vi "PythonBDConverter_String.vi"(8 "error in":errorcluster, 11 "Name":string="TestAdd.vi") -> (0 "error out":errorcluster, 3 "PythonConverter out":refnum<class "PythonBDConverter.lvclass">)   [LabVIEW 2014, in "PythonBDConverter.lvclass"]
uses:
  PythonBDConverter.lvclass
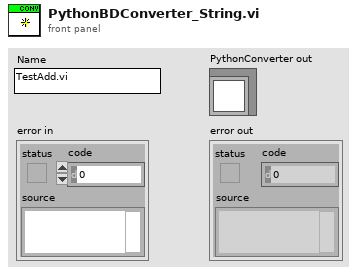
[diagram p1: front panel]
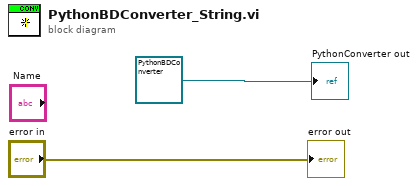
[diagram p0: block diagram]
diagram:
  "error out" <- "error in"
  "PythonConverter out" <- refnum<class "PythonBDConverter.lvclass"> refnum ("PythonConverter in")
